vi "更新程序.vi"() -> ()   [LabVIEW 2016, in "自动更新.lvlib"]
uses:
  <vilib>/FTP/NI_FTP.lvlib
panel:
  out "软件版本 2":string caption="目标软件版本"
  out "软件版本":string caption="当前软件版本"
  out "下载的文件名":string
  out "目标文件夹名":string
  out "端口号":i32
  out "IP地址":string
  out "步骤":string
  out "当前步骤":string
  in  "目标路径（使用对话框）":path
  out "下载保存目录":path
  out "更新进度":u8(slide) scale=0.0..100.0
  # "1.先下载更新-------2.关闭主应用-------3.替换应用--------4.打开主应用-----------5.关闭本程序"
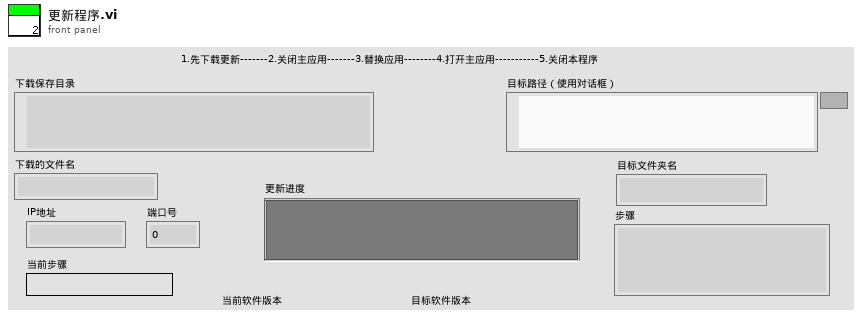
[diagram p1: front panel]
types:
  T1 = enum16{"open", "replace", "create", "open or create", "replace or create", "replace or create with confirmation"}
  T2 = cluster{"网络灯":bool, "接收中":bool, "已接收百分比":u8, "接收成功次数":dbl, "当前步骤":enum16{"init", "receivehead", "receivecontent", "receivesuccess", "over"}, "文件名":string, "error out":errorcluster}
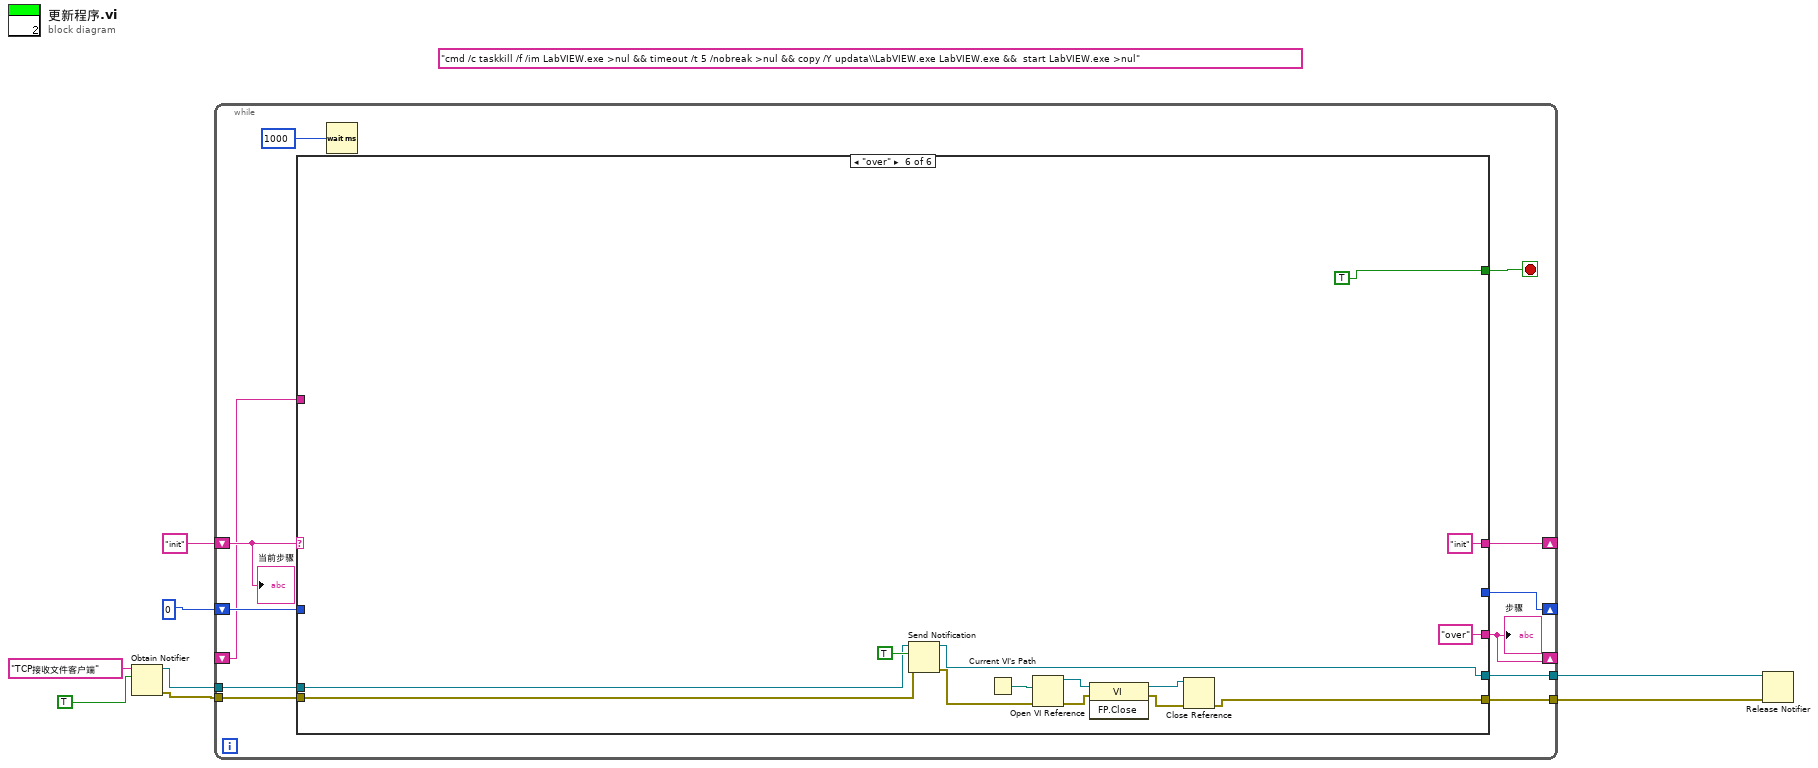
[diagram p0: block diagram]
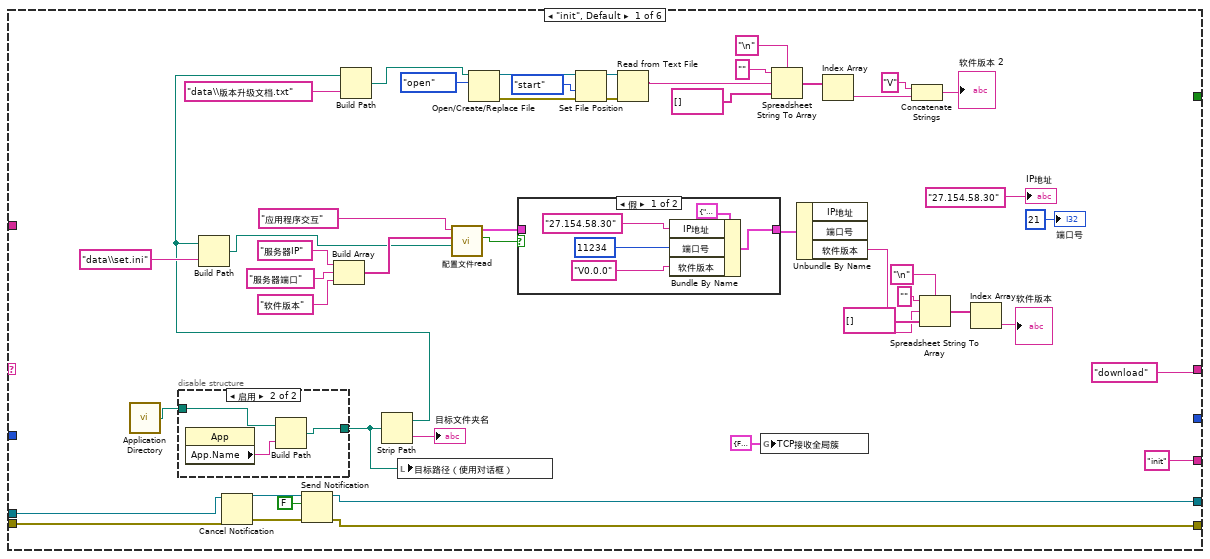
[diagram p2: hidden frame]
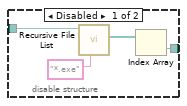
[diagram p3: hidden frame]
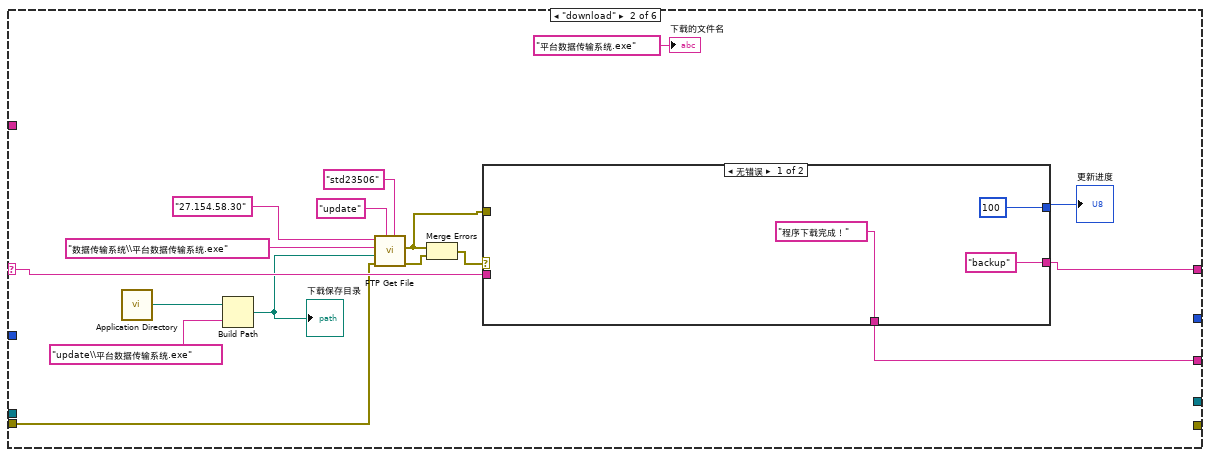
[diagram p5: hidden frame]
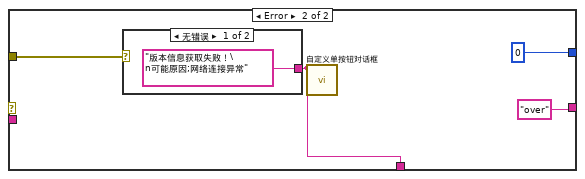
[diagram p6: hidden frame]
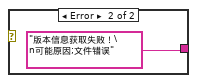
[diagram p7: hidden frame]
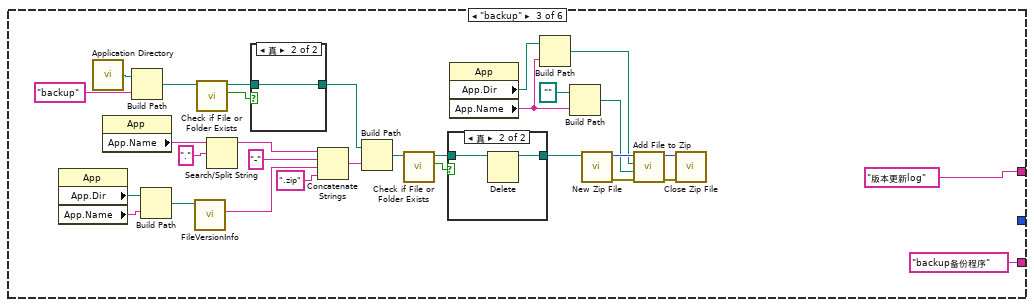
[diagram p8: hidden frame]
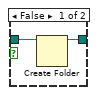
[diagram p10: hidden frame]
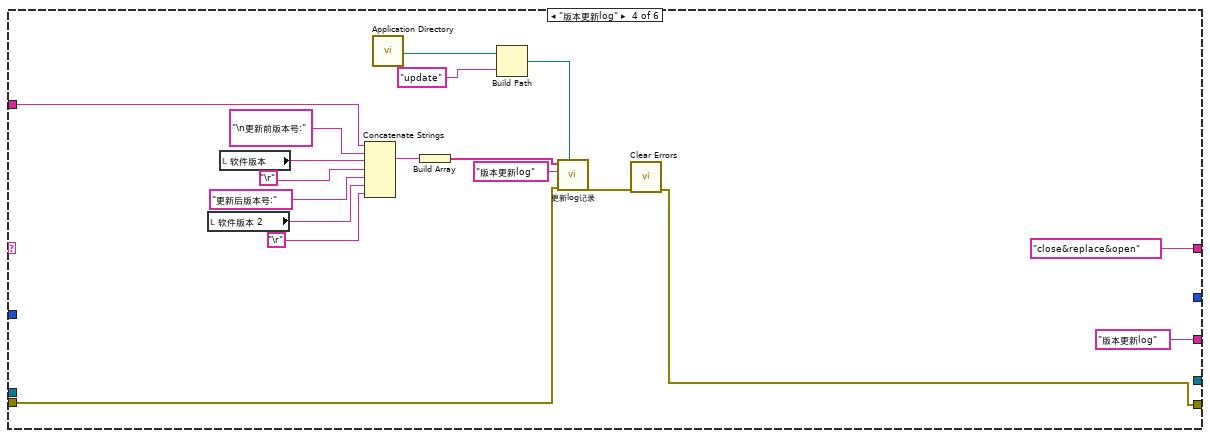
[diagram p11: hidden frame]
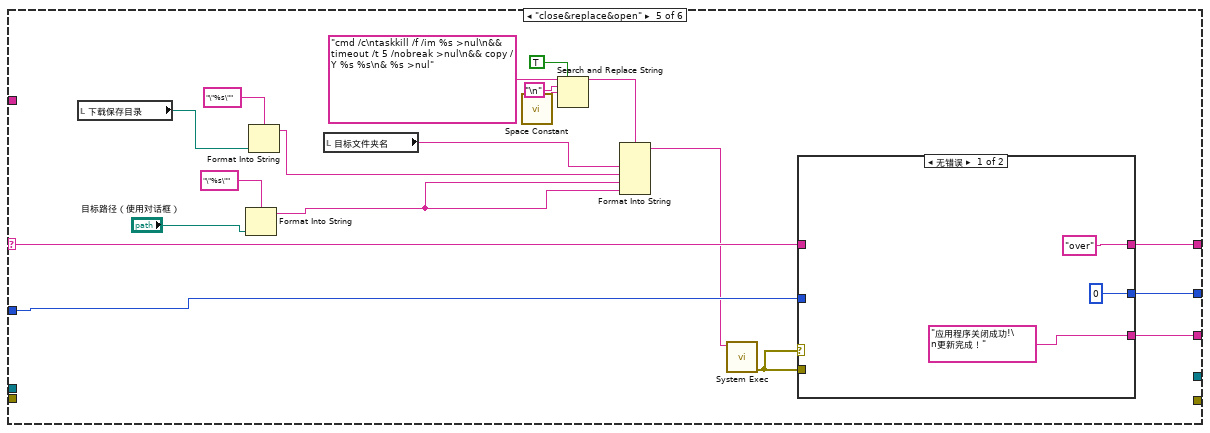
[diagram p12: hidden frame]
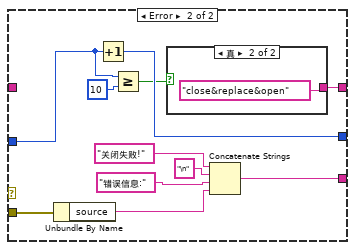
[diagram p13: hidden frame]
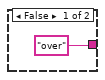
[diagram p14: hidden frame]
diagram:
  (unwired) "cmd /c taskkill /f /im LabVIEW.exe >nul && timeout /t 5 /nobreak >nul && copy /Y updata\\LabVIEW.exe LabVIEW.exe &&  start LabVIEW.exe >nul" ("结果字符串")
  n1 = Obtain Notifier(name (unnamed)="TCP接收文件客户端" ("名称（未命名）"), notification data type=TRUE) -> (notifier out=w6:refnum<notifier>, error out=w5:errorcluster)  [unwired: 2 in, 1 out]
  n2 = while {
    shift-right: [w19] -> _
    shift-left: "init" -> [w20]
    tunnel: w6 -> [w16]
    tunnel: w5 -> [w15]
    tunnel: [w14] -> w4
    tunnel: [w13] -> w3
    shift-right: [w11] -> _
    shift-left: u8 0 -> [w12]
    shift-right: [w10] -> _
    shift-left: _ -> [w9]
    stop <- w18 stop-if-true
    n3 = case shown="\"over\"" w20 {
      selector: w20 -> [_ w87 _ _ w179 _]
      tunnel: ["download" w88 "版本更新log" "close&replace&open" w178 "init"] -> w19
      tunnel: [_ _ _ _ _ TRUE] -> w18
      tunnel: ["init" ("步骤") w85 "backup备份程序" ("步骤") "版本更新log" ("步骤") w177 "over" ("步骤")] -> w10
      tunnel: w16 -> [w67 _ _ _ _ w203]
      tunnel: w15 -> [w66 w86 _ w154 _ w202]
      tunnel: [w62 _ _ _ _ w201] -> w14
      tunnel: [w61 _ _ w144 _ w200] -> w13
      tunnel: w12 -> [_ _ _ _ w176 _]
      tunnel: [_ _ _ _ w175 _] -> w11
      tunnel: w9 -> [_ _ _ w149 _ _]
      frame "init", Default {
        n4 = call <vilib>:"Application Directory.vi"() -> ("Application Directory"=w22:path)
        n5 = disable-structure shown="启用" {
          disable-tunnel: [w72 w73] -> w59
          disable-tunnel: w22 -> [w69 w75]
          frame Disabled {
            n6 = call <vilib>:"Recursive File List.vi"("pattern"="*.exe", "Folder Path"=w69) -> ("All Files in Dir"=w71:path[])  [unwired: 5 in, 4 out]
            n7 = Index Array(array=w71) -> (element=w72:path)  [unwired: 1 in]
          }
          frame Enabled {
            n8 = property class="App"() -> ("App.Name"=w74:string)  [unwired: 2 in, 2 out]
            n9 = Build Path(base path=w75, name or relative path=w74) -> (appended path=w73:path)
          }
        }
        n10 = Cancel Notification(0:w67, 3:w66) -> (8:w65:refnum<notifier>, 11:w63:errorcluster)  [unwired: 1 out]
        n11 = Send Notification(notification=FALSE ("通知"), notifier=w65, error in (no error)=w63) -> (notifier out=w62:refnum<notifier>, error out=w61:errorcluster)
        n12 = Build Array("服务器IP" ("section"), "服务器端口" ("section"), "软件版本" ("key")) -> (w31:string[])
        n13 = Strip Path(path=w59) -> (stripped path=w35:path, name=→"目标文件夹名":string)
        n14 = Build Path(base path=w35, name or relative path="data\\set.ini" ("名称或相对路径")) -> (appended path=w27:path)
        n15 = Build Path(base path=w35, name or relative path="data\\版本升级文档.txt" ("名称或相对路径")) -> (appended path=w43:path)
        n16 = local write "目标路径（使用对话框）"(w59) -> ()
        n17 = call "配置文件read.vi"("configuration file path"=w27, "键数组"=w31, "段"="应用程序交互" ("section")) -> ("section exists?"=w33:bool, "updateconfiguration"=w34:cluster{"IP地址":string, "端口号":i32, "软件版本":string})  [unwired: 6 in, 1 out]
        n18 = Open/Create/Replace File(file path (use dialog)=w43, operation (0:open)=T1."open" ("操作(0:open)")) -> (refnum out=w38:refnum<file>, error out=w39:errorcluster)  [unwired: 4 in, 1 out]
        n19 = case shown="假" w33 {
          tunnel: w34 -> [_ w81]
          tunnel: [w76 w81] -> w26
          frame False {
            n20 = Bundle By Name(cluster=cluster{"IP地址":string, "端口号":i32, "软件版本":string} {"IP地址"="", "端口号"=0, "软件版本"=""} ("updateconfiguration"), "IP地址"="27.154.58.30" ("key"), "端口号"=11234 ("value"), "软件版本"="V0.0.0" ("key")) -> (w76:cluster{"IP地址":string, "端口号":i32, "软件版本":string})
          }
          frame True {
          }
        }
        n21 = Set File Position(refnum=w38, from (0:start)=enum16{"start", "end", "current"}."start" ("自（0:起始）"), error in=w39) -> (refnum out=w42:refnum<file>, error out=w40:errorcluster)  [unwired: 1 in]
        n22 = Read from Text File(file (use dialog)=w42, error in=w40) -> (text=w50:string)  [unwired: 2 in, 3 out]
        n23 = global write "全局变量1.vi" "TCP接收全局簇"(T2 {"网络灯"=FALSE, "接收中"=FALSE, "已接收百分比"=0, "接收成功次数"=0.0, "当前步骤"=enum."init", "文件名"="", "error out"={"status"=FALSE, "code"=0, "source"=""}} ("TCP接收全局簇")) -> ()
        n24 = Spreadsheet String To Array(delimiter (Tab)="\n" ("分隔符(Tab)"), format string="" ("格式字符串"), spreadsheet string=w50, array type (2D Dbl)=string[] []) -> (array=w47:string[])
        n25 = Unbundle By Name(w26) -> ("软件版本"=w25:string)  [unwired: 2 out]
        n26 = Index Array(array=w47) -> (element=w48:string)  [unwired: 1 in]
        n27 = Concatenate Strings("V" ("字符串"), w48) -> (→"软件版本 2":string)
        n28 = Spreadsheet String To Array(delimiter (Tab)="\n" ("分隔符(Tab)"), format string="" ("格式字符串"), spreadsheet string=w25, array type (2D Dbl)=string[] []) -> (array=w53:string[])
        n29 = Index Array(array=w53) -> (element=→"软件版本":string)  [unwired: 1 in]
        "IP地址" <- "27.154.58.30" ("key")
        "端口号" <- 21 ("端口号")
      }
      frame "download" {
        n30 = call <vilib>:"Application Directory.vi"() -> ("Application Directory"=w82:path)
        n31 = Build Path(base path=w82, name or relative path="update\\平台数据传输系统.exe" ("名称或相对路径")) -> (appended path=w83:path)
        "下载保存目录" <- w83
        n32 = call <vilib>:"FTP Get File.vi"("password"="std23506", "user"="update", "error in (no error)"=w86, "local path"=w83, "remote path"="数据传输系统\\平台数据传输系统.exe", "host"="27.154.58.30") -> ("error out"=w93:errorcluster, "file error"=w92:errorcluster)  [unwired: 4 in]
        n33 = Merge Errors(w92, w93) -> (w91:errorcluster)
        n34 = case shown="无错误" w91 {
          tunnel: w92 -> [_ w104]
          tunnel: [u8 100 ("y") u8 0 ("y")] -> w90
          tunnel: ["backup" "over"] -> w88
          tunnel: w87 -> [_ _]
          tunnel: ["程序下载完成！" w102] -> w85
          frame No Error {
          }
          frame Error {
            n35 = case shown="无错误" w104 {
              tunnel: ["版本信息获取失败！\n可能原因;网络连接异常" "版本信息获取失败！\n可能原因;文件错误"] -> w102
              frame No Error {
              }
              frame Error {
              }
            }
            n36 = call "自定义单按钮对话框.vi"("消息"=w102) -> ()  [unwired: 11 in]
          }
        }
        "更新进度" <- w90
        "下载的文件名" <- "平台数据传输系统.exe" ("下载的文件名")
      }
      frame "backup" {
        n37 = property class="App"() -> ("App.Dir"=w129:path, "App.Name"=w135:string)  [unwired: 2 in, 2 out]
        n38 = call <vilib>:"Application Directory.vi"() -> ("Application Directory"=w136:path)
        n39 = property class="App"() -> ("App.Name"=w133:string)  [unwired: 2 in, 2 out]
        n40 = Build Path(base path=w136, name or relative path="backup" ("名称或相对路径")) -> (appended path=w116:path)
        n41 = Build Path(base path=w129, name or relative path=w135) -> (appended path=w134:path)
        n42 = call <vilib>:"FileVersionInfo.vi"("Application Path in"=w134) -> ("File Version Info"=w131:string)  [unwired: 7 in, 3 out]
        n43 = call <vilib>:"Check if File or Folder Exists.vi"("path"=w116) -> ("file or folder exists?"=w115:bool, "dup path"=w114:path)  [unwired: 8 in, 1 out]
        n44 = Search/Split String(string=w133, search string/char (-)="." ("搜索字符串/字符(-)")) -> (substring before match=w127:string)  [unwired: 1 in, 2 out]
        n45 = case shown="真" w115 {
          tunnel: w114 -> [w142 w143]
          tunnel: [w141 w143] -> w113
          frame False {
            n46 = Create Folder(path (use dialog)=w142) -> (created path=w141:path)  [unwired: 2 in, 2 out]
          }
          frame True {
          }
        }
        n47 = Concatenate Strings(w127, "-" ("字符串"), w131, ".zip" ("字符串")) -> (w126:string)
        n48 = Build Path(base path=w113, name or relative path=w126) -> (appended path=w110:path)
        n49 = call <vilib>:"Check if File or Folder Exists.vi"("path"=w110) -> ("file or folder exists?"=w111:bool, "dup path"=w112:path)  [unwired: 8 in, 1 out]
        n50 = case shown="真" w111 {
          tunnel: w112 -> [w138 w140]
          tunnel: [w138 w139] -> w109
          frame False {
          }
          frame True {
            n51 = Delete(path (use dialog)=w140) -> (deleted path=w139:path)  [unwired: 4 in, 2 out]
          }
        }
        n52 = property class="App"() -> ("App.Dir"=w125:path, "App.Name"=w118:string)  [unwired: 2 in, 2 out]
        n53 = Build Path(base path=w125, name or relative path=w118) -> (appended path=w120:path)
        n54 = Build Path(base path=path "" ("Relative Path from 1 to 2"), name or relative path=w118) -> (appended path=w117:path)
        n55 = call <vilib>:"New Zip File.vi"("target"=w109) -> ("error out"=w124:errorcluster, "zip file out"=w123:i64)  [unwired: 2 in, 3 out]
        n56 = call <vilib>:"Add File to Zip.vi"("error in (no error)"=w124, "destination path in zip"=w117, "source file path"=w120, "zip file in"=w123) -> ("error out"=w121:errorcluster, "zip file out"=w122:i64)  [unwired: 6 in]
        n57 = call <vilib>:"Close Zip File.vi"("error in (no error)"=w121, "zip file in"=w122) -> ()  [unwired: 5 in, 1 out]
      }
      frame "版本更新log" {
        n58 = local read "软件版本 2"() -> (w151:string)
        n59 = local read "软件版本"() -> (w153:string)
        n60 = Concatenate Strings(w149, "\n更新前版本号:" ("字符串"), w153, "\r", "更新后版本号:", w151, "\r") -> (w159:string)
        n61 = call <vilib>:"Application Directory.vi"() -> ("Application Directory"=w147:path)
        n62 = Build Array(w159) -> (w158:string[])
        n63 = Build Path(base path=w147, name or relative path="update" ("名称或相对路径")) -> (appended path=w146:path)
        n64 = call "更新log记录.vi"("路径"=w146, "错误输入（无错误）"=w154, "logname"="版本更新log", "数组"=w158) -> ("错误输出"=w155:errorcluster)  [unwired: 7 in]
        n65 = call <vilib>:"Clear Errors.vi"("error in (no error)"=w155) -> ("error out"=w144:errorcluster)  [unwired: 5 in, 1 out]
      }
      frame "close&replace&open" {
        n66 = local read "下载保存目录"() -> (w167:path)
        n67 = Format Into String(format string="\"%s\"" ("格式字符串"), "目标路径（使用对话框）") -> (resulting string=w163:string)  [unwired: 2 in, 1 out]
        n68 = Format Into String(format string="\"%s\"" ("格式字符串"), w167) -> (resulting string=w165:string)  [unwired: 2 in, 1 out]
        n69 = local read "目标文件夹名"() -> (w174:string)
        n70 = call <vilib>:"Space Constant.vi"() -> ("String"=w170:string)
        n71 = Search and Replace String(replace all?=TRUE ("替换全部？(F)"), input string="cmd /c\ntaskkill /f /im %s >nul\n&& timeout /t 5 /nobreak >nul\n&& copy /Y %s %s\n& %s >nul" ("名称或相对路径"), search string="\n", replace string=w170) -> (result string=w173:string)  [unwired: 4 in, 3 out]
        n72 = Format Into String(format string=w173, w174, w165, w163, w163) -> (resulting string=w168:string)  [unwired: 2 in, 1 out]
        n73 = call <vilib>:"System Exec.vi"("command line"=w168) -> ("error out"=w180:errorcluster)  [unwired: 7 in, 3 out]
        n74 = case shown="无错误" w180 {
          tunnel: ["over" w188] -> w178
          tunnel: w180 -> [_ w194]
          tunnel: ["应用程序关闭成功!\n更新完成！" ("步骤") w189] -> w177
          tunnel: w179 -> [_ _]
          tunnel: w176 -> [_ w184]
          tunnel: [u8 0 w186] -> w175
          frame No Error {
          }
          frame Error {
            n75 = Unbundle By Name(w194) -> ("source"=w193:string)
            n76 = Increment(x=w184) -> (x+1=w186:u8)
            n77 = Greater Or Equal?(x=w184, y=u8 10) -> (x >= y?=w185:bool)
            n78 = case shown="真" w185 {
              tunnel: ["over" "close&replace&open"] -> w188
              frame False {
              }
              frame True {
              }
            }
            n79 = Concatenate Strings("关闭失败!" ("消息"), "\n" ("字符串"), "错误信息:" ("字符串"), w193) -> (w189:string)
          }
        }
      }
      frame "over" {
        n80 = Send Notification(notification=TRUE, notifier=w203, error in (no error)=w202) -> (notifier out=w201:refnum<notifier>, error out=w206:errorcluster)
        n81 = Current VI's Path() -> (path=w208:path)
        n82 = Open VI Reference(vi path=w208, error in (no error)=w206) -> (vi reference=w207:refnum<vi>, error out=w209:errorcluster)  [unwired: 4 in]
        n83 = invoke class="VI" method="FP.Close"(reference=w207, error in=w209) -> (reference out=w204:refnum<vi>, error out=w205:errorcluster)  [unwired: 1 in, 1 out]
        n84 = Close Reference(reference=w204, error in (no error)=w205) -> (error out=w200:errorcluster)
      }
    }
    "步骤" <- w10
    n85 = Wait (ms)(milliseconds to wait=u32 1000 ("等待时间（毫秒）")) -> ()  [unwired: 1 out]
    "当前步骤" <- w20
  }
  n86 = Release Notifier(notifier=w4, error in (no error)=w3) -> ()  [unwired: 1 in, 3 out]
